vi "ElevatorSim_Rkf45_Func.vi"(9 "U":T1, 10 "X":T1, 11 "Variant":variant) -> (0 "Error":bool, 3 "NewX":T1)   [LabVIEW 2019, in "Trajectory_Library.lvlib"]
uses:
  Trajectory_Library.lvlib
  <vilib>/Analysis/Matrix/Datatypes/RealMatrix.ctl
  <vilib>/Analysis/baseanly.llb/Real A x B.vi
  <vilib>/Analysis/Matrix/Numeric/Add/Add - RM,RM.vi
  <vilib>/Analysis/Matrix/NI_Matrix.lvlib
  <vilib>/Analysis/NI_AALBase.lvlib
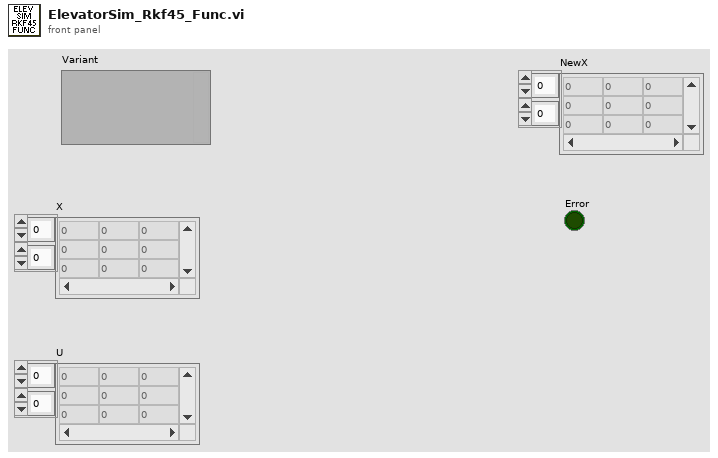
[diagram p1: front panel]
types:
  T1 = typedef "NI_Matrix.lvlib/RealMatrix.ctl" = dbl[][]
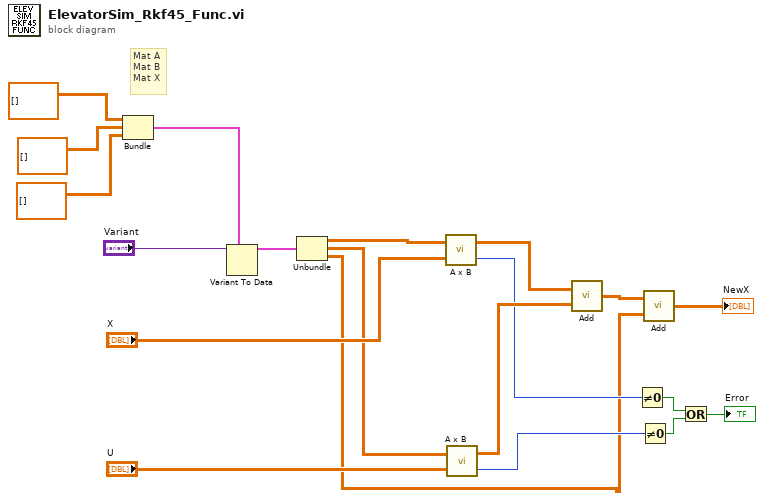
[diagram p0: block diagram]
diagram:
  # "Mat A\nMat B\nMat X"
  n1 = Bundle("matrix"=T1 [], "matrix"=T1 [], "matrix"=T1 []) -> (w16:cluster{"matrix":T1, "matrix":T1, "matrix":T1})  [unwired: 1 in]
  n2 = Variant To Data(type=w16, Variant="Variant") -> (data=w15:cluster{"matrix":T1, "matrix":T1, "matrix":T1})  [unwired: 1 in, 1 out]
  n3 = Unbundle(w15) -> ("matrix"=w7:T1, "matrix"=w5:T1, "matrix"=w3:T1)
  n4 = call-poly <vilib>:"A x B.vi"("B"="X", "A"=w7) -> ("error"=w9:i32, "A x B"=w14:T1)
  n5 = call-poly <vilib>:"A x B.vi"("B"="U", "A"=w5) -> ("error"=w8:i32, "A x B"=w13:T1)
  n6 = call-poly <vilib>:"Add.vi"("Real Matrix B"=w13, "Real Matrix A"=w14) -> ("A + B"=w12:T1)
  n7 = Not Equal To 0?(x=w9) -> (x != 0?=w11:bool)
  n8 = Not Equal To 0?(x=w8) -> (x != 0?=w10:bool)
  n9 = call-poly <vilib>:"Add.vi"("Real Matrix B"=w3, "Real Matrix A"=w12) -> ("A + B"=→"NewX":T1)
  n10 = Or(x=w11, y=w10) -> (x .or. y?=→"Error":bool)
